vi "Measure.vi"(8 "error in":errorcluster, 11 "Instrument Driver in":refnum<class "Instrument Driver.lvclass">) -> (0 "error out":errorcluster, 2 "Measurement Results":T1={"Voltage (V)"=1.0} {"Voltage (V)" min=-424.2 max=424.2 step=1.0 format="%#.1f"}, 3 "Instrument Driver out":refnum<class "Instrument Driver.lvclass">)   [LabVIEW 2020, in "Plugin Instrument Driver.lvlib" / "Instrument Driver.lvclass"]
doc: "Reads the Measurement."
uses:
  Instrument Driver.lvclass
  Typedefs/Measurement Results.ctl
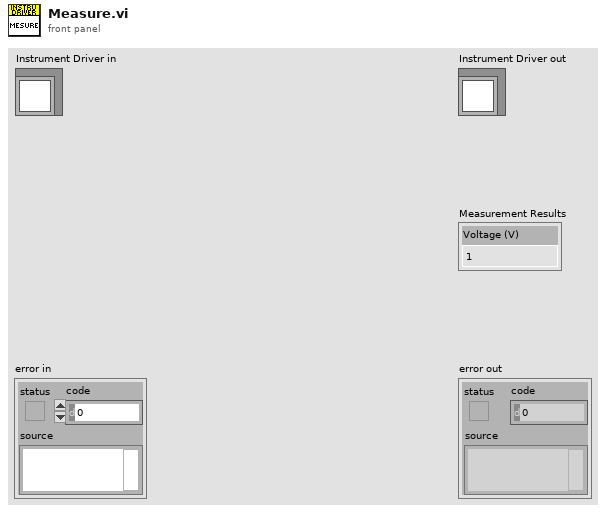
[diagram p1: front panel]
types:
  T1 = typedef "Plugin Instrument Driver.lvlib/Instrument Driver.lvclass/Measurement Results.ctl" = cluster{"Voltage (V)":dbl}
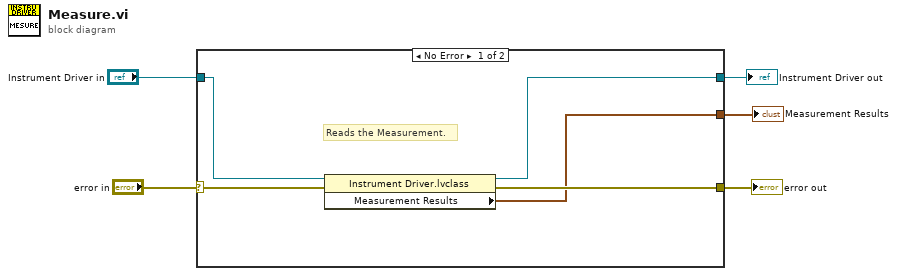
[diagram p0: block diagram]
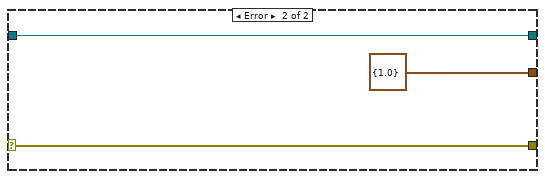
[diagram p2: hidden frame]
diagram:
  n1 = case shown="No Error" "error in" {
    selector: "error in" -> [w8 w13]
    tunnel: [w7 w13] -> w4
    tunnel: [w9 w12] -> w2
    tunnel: "Instrument Driver in" -> [w10 w12]
    tunnel: [w6 T1 {"Voltage (V)"=1.0} ("Measurement Results")] -> w1
    frame No Error {
      # "Reads the Measurement."
      n2 = property class="Instrument Driver.lvclass"(reference=w10, error in=w8) -> (reference out=w9:refnum<class "Instrument Driver.lvclass">, error out=w7:errorcluster, "Measurement Results"=w6:T1)
    }
    frame Error {
    }
  }
  "error out" <- w4
  "Instrument Driver out" <- w2
  "Measurement Results" <- w1
